vi "checkBeginStopOffensivePlay.vi"(8 "error in (no error)":errorcluster, 10 "Game":refnum<class "Game.lvclass">, 11 "StopOffensivePlay in":refnum<class "StopOffensivePlay.lvclass">) -> (0 "error out":errorcluster, 2 "Boolean":bool, 3 "StopOffensivePlay out":refnum<class "StopOffensivePlay.lvclass">)   [LabVIEW 2023, in "StopOffensivePlay.lvclass"]
uses:
  StopOffensivePlay.lvclass
  Game_class/Game.lvclass
  Referee_class/command_interpreted.ctl
  Game_class/Game.lvclass/Game.ctl
  Referee_class/Referee.lvclass/Referee.ctl
  Events_class/Events.lvclass/Events.ctl
  Game_class/Read Referee.vi
  Game_class/Read EventsRef.vi
  Events_class/Read ball_out.vi
  Referee_class/Read command_interpreted.vi
  Referee_class/Referee.lvclass
  Events_class/Events.lvclass
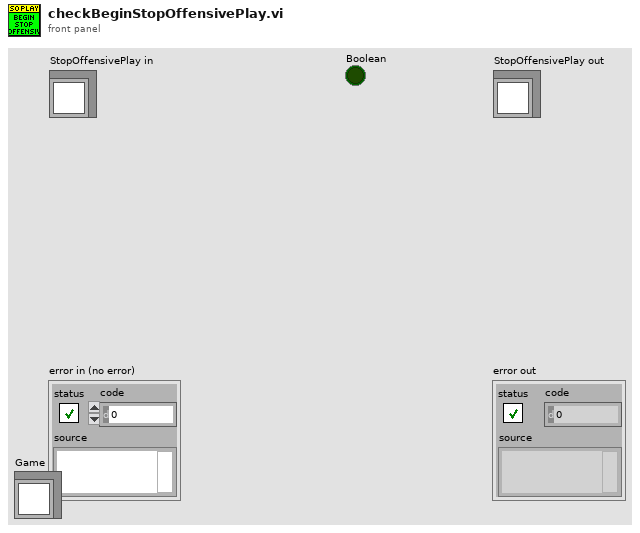
[diagram p1: front panel]
types:
  T1 = typedef "command_interpreted.ctl" = enum16{"Goal Ally", "Goal Enemy", "Ball Placement Enemy", "Ball Placement Ally", "Normal Half Time", "Extra Time  Break", "Extra Half Time", "None", "Post Game", "PKA Normal Start", "Prepare Kickoff Ally", "PKE Normal Start", "Prepare Kickoff Enemy", "Force Start", "Halt", "Timeout", "Prepare Penalty Ally", "Prepare Penalty Enemy", "PPA NormalStart", "PPE Normal Start", "Indirect Free Ally", "Direct Free Enemy", "Direct Free Ally", "Indirect Free Enemy", "Stop"}
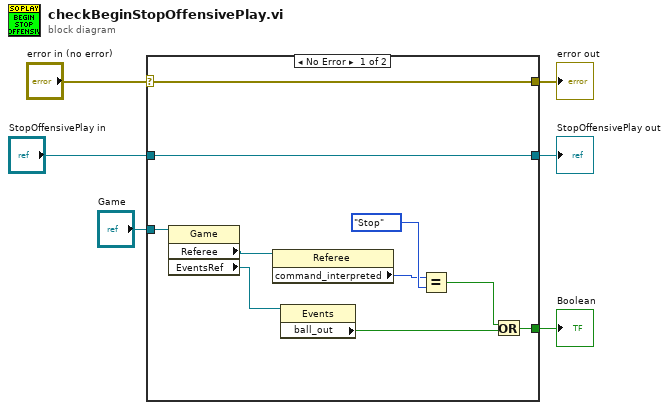
[diagram p0: block diagram]
diagram:
  n1 = case shown="No Error" "error in (no error)" {
    selector: "error in (no error)" -> [w15 w18]
    tunnel: [w15 w18] -> w5
    tunnel: [w16 w17] -> w3
    tunnel: "StopOffensivePlay in" -> [w16 w17]
    tunnel: "Game" -> [w11 _]
    tunnel: [w8 _] -> w1
    frame No Error {
      n2 = property class="Game"(reference=w11) -> ("Referee"=w14:refnum<class "Referee.lvclass">, "EventsRef"=w10:refnum<class "Events.lvclass">)  [unwired: 1 in, 2 out]
      n3 = property class="Referee"(reference=w14) -> ("command_interpreted"=w12:T1)  [unwired: 1 in, 2 out]
      n4 = property class="Events"(reference=w10) -> ("ball_out"=w9:bool)  [unwired: 1 in, 2 out]
      n5 = Equal?(x=w12, y=command_interpreted."Stop" ("command_interpreted")) -> (x = y?=w7:bool)
      n6 = Or(x=w7, y=w9) -> (x .or. y?=w8:bool)
    }
    frame Error {
    }
  }
  "error out" <- w5
  "StopOffensivePlay out" <- w3
  "Boolean" <- w1
